vi "hours between scans.vi"(9 "Number of hours To Collect before starting new file":u16 min=1 max=24 step=1, 11 "Input start time":dbl) -> (0 "error out":errorcluster, 1 "Time has Elapsed":bool, 3 "output next start time":dbl)   [LabVIEW 2009]
uses:
  <vilib>/Utility/miscctls.llb/LVDateTimeRec.ctl
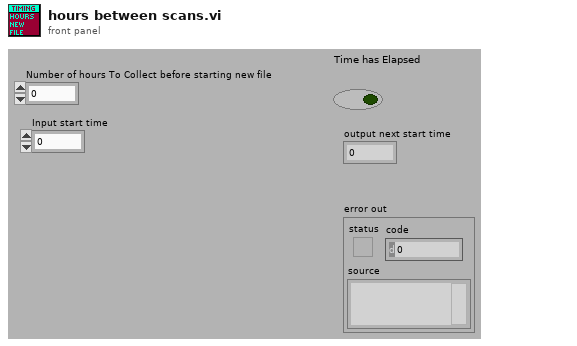
[diagram p1: front panel]
types:
  T1 = typedef "LVDateTimeRec.ctl" = cluster{"fractional second":dbl, "second":i32, "minute":i32, "hour":i32, "day of month":i32, "month":i32, "year":i32, "day of week":i32, "day of year":i32, "DST":i32}
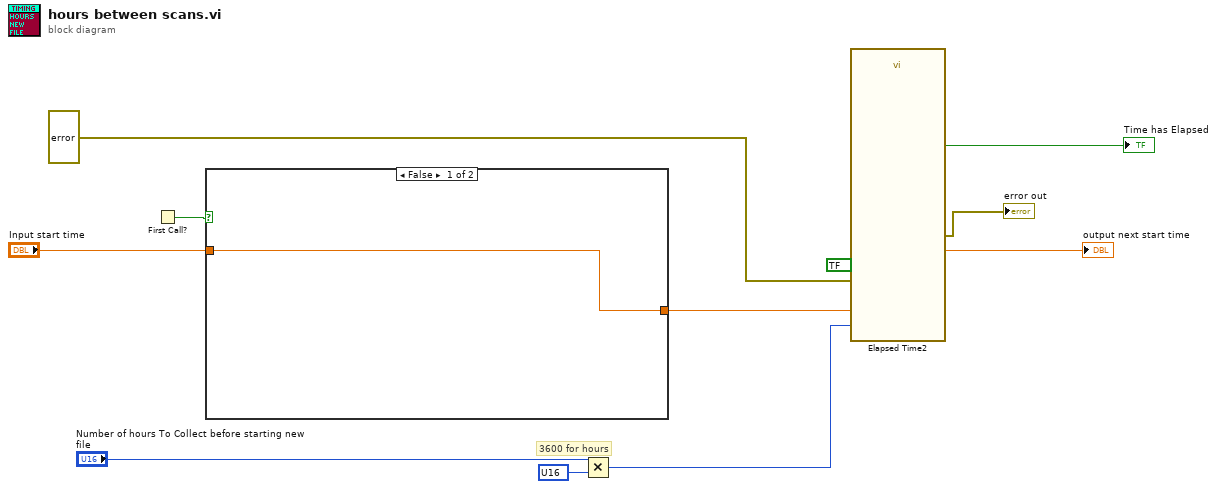
[diagram p0: block diagram]
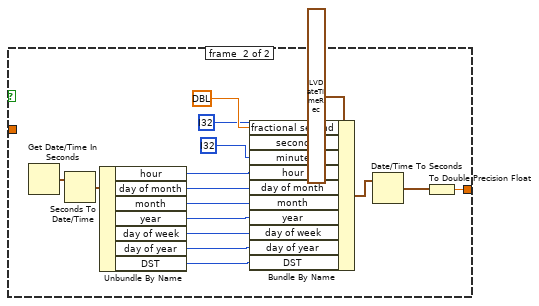
[diagram p2: hidden frame]
diagram:
  # "3600 for hours"
  n1 = First Call?() -> (First Call?: T/F=w1:bool)
  n2 = case shown="False" w1 {
    tunnel: [w12 w13] -> w4
    tunnel: "Input start time" -> [w12 _]
    frame #0 {
    }
    frame #1 {
      n3 = Get Date/Time In Seconds() -> (seconds since 1Jan1904=w19:timestamp)
      n4 = Seconds To Date/Time(time stamp (now)=w19) -> (date time rec=w18:T1)  [unwired: 1 in]
      n5 = Unbundle By Name(w18) -> ("hour"=w15:i32, "day of month"=w20:i32, "month"=w27:i32, "year"=w26:i32, "day of week"=w25:i32, "day of year"=w24:i32, "DST"=w23:i32)
      n6 = Bundle By Name(cluster=T1 ? ("date time rec 2"), "fractional second"=dbl ?, "second"=i32 ?, "minute"=i32 ?, "hour"=w15, "day of month"=w20, "month"=w27, "year"=w26, "day of week"=w25, "day of year"=w24, "DST"=w23) -> (w21:T1)
      n7 = Date/Time To Seconds(2:w21) -> (0:w14:timestamp)  [unwired: 1 in]
      n8 = To Double Precision Float(number=w14) -> (double precision float=w13:dbl)
    }
  }
  n9 = Multiply(x="Number of hours To Collect before starting new file", y=u16 ?) -> (x*y=w3:u16)
  n10 = call "Elapsed Time2"("Time Target (s)"=w3, "Auto Reset"=bool ?, "error in (no error)"=errorcluster ?, "Set Start Time (s)"=w4) -> ("Get Start Time (s)"=→"output next start time":dbl, "Time has Elapsed"=→"Time has Elapsed":bool, "error out"=→"error out":errorcluster)  [unwired: 8 in, 5 out]
